vi "clickInsideImage.vi"(8 "error in (no error)":errorcluster, 10 "Point":T1, 11 "ImageStreamViewer in":refnum<class "ImageStreamViewer.lvclass">) -> (0 "error out":errorcluster, 2 "clickInsideImage?":bool, 3 "ImageStreamViewer out":refnum<class "ImageStreamViewer.lvclass">)   [LabVIEW 2009, in "Views.lvlib" / "Camera.lvlib" / "ImageStreamViewer.lvclass"]
uses:
  ImageStreamViewer.lvclass
  <vilib>/Utility/miscctls.llb/LVPoint32TypeDef.ctl
  ImageStreamViewer.lvclass/ImageStreamViewer.ctl
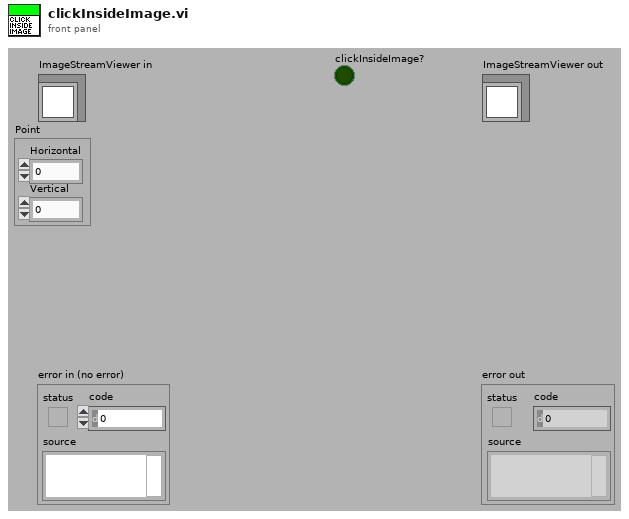
[diagram p1: front panel]
types:
  T1 = typedef "LVPoint32TypeDef.ctl" = cluster{"Horizontal":i32, "Vertical":i32}
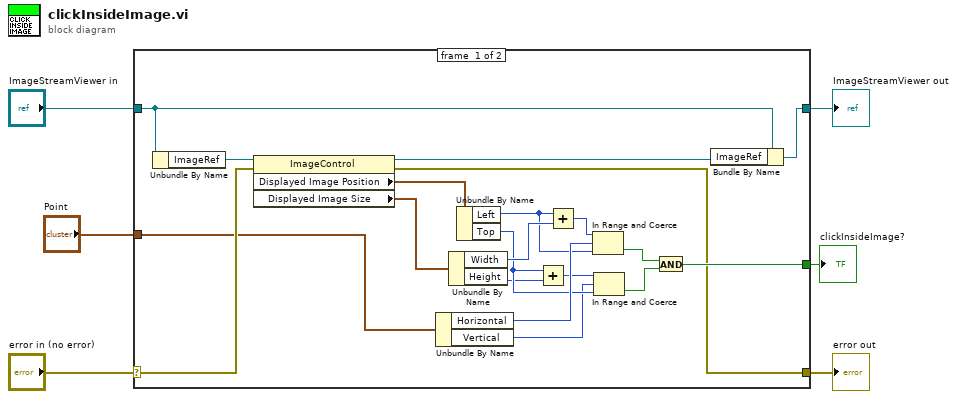
[diagram p0: block diagram]
diagram:
  n1 = case shown="No Error" "error in (no error)" {
    selector: "error in (no error)" -> [w25 w28]
    tunnel: [w8 w28] -> w5
    tunnel: [w9 w27] -> w3
    tunnel: "ImageStreamViewer in" -> [w10 w27]
    tunnel: [w12 _] -> w2
    tunnel: "Point" -> [w7 _]
    frame #0 {
      n2 = Unbundle By Name(w10) -> ("ImageRef"=w26:refnum<vi>)
      n3 = property class="ImageControl"(reference=w26, error in=w25) -> (reference out=w11:refnum<vi>, error out=w8:errorcluster, "Displayed Image Position"=w24:cluster{"Left":i32, "Top":i32}, "Displayed Image Size"=w23:cluster{"Width":u32, "Height":u32})
      n4 = Unbundle By Name(w7) -> ("Horizontal"=w22:i32, "Vertical"=w15:i32)
      n5 = Unbundle By Name(w23) -> ("Width"=w20:u32, "Height"=w16:u32)
      n6 = Unbundle By Name(w24) -> ("Left"=w19:i32, "Top"=w17:i32)
      n7 = Add(x=w17, y=w16) -> (x+y=w18:u32)
      n8 = Add(x=w19, y=w20) -> (x+y=w21:u32)
      n9 = In Range and Coerce(upper limit=w21, x=w22, lower limit=w19) -> (In Range?=w14:bool)  [unwired: 1 out]
      n10 = In Range and Coerce(upper limit=w18, x=w15, lower limit=w17) -> (In Range?=w13:bool)  [unwired: 1 out]
      n11 = And(x=w14, y=w13) -> (x .and. y?=w12:bool)
      n12 = Bundle By Name(cluster=w10, "ImageRef"=w11) -> (w9:refnum<class "ImageStreamViewer.lvclass">)
    }
    frame #1 {
    }
  }
  "error out" <- w5
  "ImageStreamViewer out" <- w3
  "clickInsideImage?" <- w2
